vi "AbsolutePlungerPosition (SubVI).vi"(11 "VISA Refnum in":refnum<visa-resource-name>) -> (3 "Plunger Position":i32)   [LabVIEW 2020]
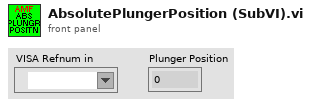
[diagram p1: front panel]
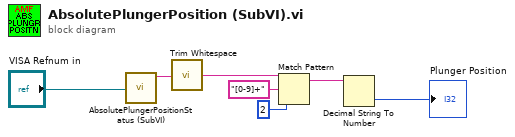
[diagram p0: block diagram]
diagram:
  n1 = call "AbsolutePlungerPositionStatus (SubVI).vi"("VISA Refnum in"="VISA Refnum in") -> ("read buffer"=w2:string)  [unwired: 10 in]
  n2 = call <vilib>:"Trim Whitespace.vi"("string"=w2) -> ("trimmed string"=w5:string)  [unwired: 1 in]
  n3 = Match Pattern(string=w5, regular expression="[0-9]+", offset (0)=2) -> (match substring=w6:string)  [unwired: 3 out]
  n4 = Decimal String To Number(string=w6) -> (number=→"Plunger Position":i32)  [unwired: 2 in, 1 out]
